vi "MesaurementType.vi"() -> ()   [LabVIEW 2011]
panel:
  in  "mesaurement type":enum32{"Point", "Area"}(radio)
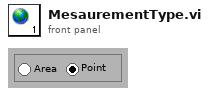
[diagram p1: front panel]
diagram:
